vi "tsdiag_can_write_data_by_identifier.vi"(6 "Data":u8[](array[numeric]), 8 "error in (no error)":errorcluster, 9 "ADataIdentifier":u16 format="%.0x", 10 "ADiagModuleIndex":i32, 11 "路径输入":path) -> (0 "error out":errorcluster, 2 "return":i32, 3 "路径输出":path)   [LabVIEW 2014]
doc: "2E服务，根据ID写入数据。"
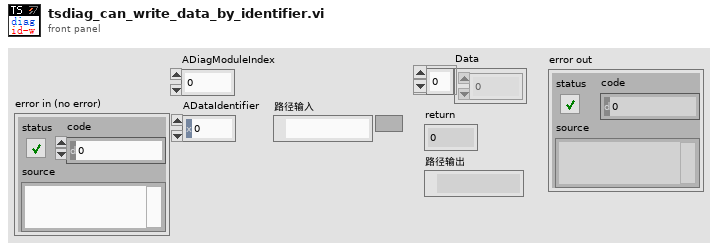
[diagram p1: front panel]
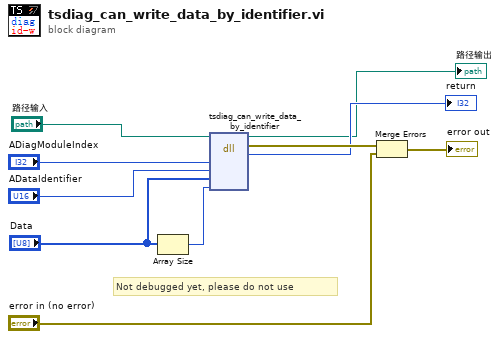
[diagram p0: block diagram]
diagram:
  # "Not debugged yet, please do not use"
  n1 = Array Size(array="Data") -> (size(s)=w5:i32)
  n2 = dll-call lib="D:/Program Files (x86)/TOSUN/TSMaster/bin/TSMaster.dll" fn="tsdiag_can_write_data_by_identifier"(path in="路径输入", "ADiagModuleIndex"="ADiagModuleIndex", "ADataIdentifier"="ADataIdentifier", "AWriteData"="Data", "AWriteDataSize"=w5) -> (path out=→"路径输出":path, error out=w10:errorcluster, "ACode"=→"return":i32)  [unwired: 6 in]
  n3 = Merge Errors(w10, "error in (no error)") -> (→"error out":errorcluster)
